vi "Tip Shaper_plus_plus.vi"() -> ()   [LabVIEW 2014]
doc: "Performs a configurable bias/Z sequence that can help to shape a STM tip.\n\n- Nanonis Programming Interface -"
uses:
  <userlib>/Nanonis Prog Interface V5/Nanonis Prog Interface.lvlib
panel:
  in  "Clear Markers":bool
  in  "Current Gain":u16(ring)=13 items=["HS 10^5", "HS 10^6", "HS 10^7", "HS 10^8", "HS 10^9", "HS 10^10", "HS 10^11", "LN 10^3", "LN 10^4", "LN 10^5", "LN 10^6", "LN 10^7", "LN 10^8", "LN 10^9"]
  in  "Bias value":dbl=0.02 format="%.3p"
  in  "Change Bias":bool=TRUE
  in  "Switch Gain":bool=TRUE
  in  "Draw":bool=TRUE
  in  "Lift Time 1":dbl=0.2 min=0.02 max=600.0 format="%.2p"
  out "Bias (V)":sgl=-2.0 format="%_5p"
  in  "Feedback":bool=TRUE
  out "oStartSequence":refnum<k4>
  in  "cleanTip":bool
  out "allQuit":bool=TRUE
  in  "quit":bool=TRUE
  out "oUpdateDisplay":refnum<k4>
  in  "End Wait Time":dbl=0.1 format="%.2p"
  in  "Lifting Bias":dbl=2.0 format="%.3p"
  in  "Lift Time 2":dbl=1.0 min=0.02 max=600.0 format="%.2p"
  in  "Lift Height":dbl=5e-09 format="%.2p"
  in  "Switch Off Delay":dbl=0.05 format="%.2p"
  in  "Bias Settling Time":dbl=0.09999999999999999 format="%.2p"
  in  "TipLift":dbl=-2e-10 format="%.2p"
  out "Z Graph":cluster{dbl[], dbl[]}[](graph)=[{[0.0, 0.10999999999999999, 0.10999999999999999, 0.20999999999999996, 0.41, 0.41, 0.51, 1.51, 1.51, 1.61], [0.0, 0.0, 0.0, 0.0, -2e-10, -2e-10, -2e-10, 5e-09, 5e-09, 5e-09]}, {[0.0, 0.10999999999999999, 0.10999999999999999, 0.20999999999999996, 0.41, 0.41, 0.51, 1.51, 1.51, 1.61], [-2.0, -2.0, 1.0, 1.0, 1.0, 2.0, 2.0, 2.0, -2.0, -2.0]}]
  # "Parameters"
  # "Internal Variables"
  # "s"
  # "V"
  # "m"
  # "s"
  # "V"
  # "s"
  # "m"
  # "s"
  # "s"
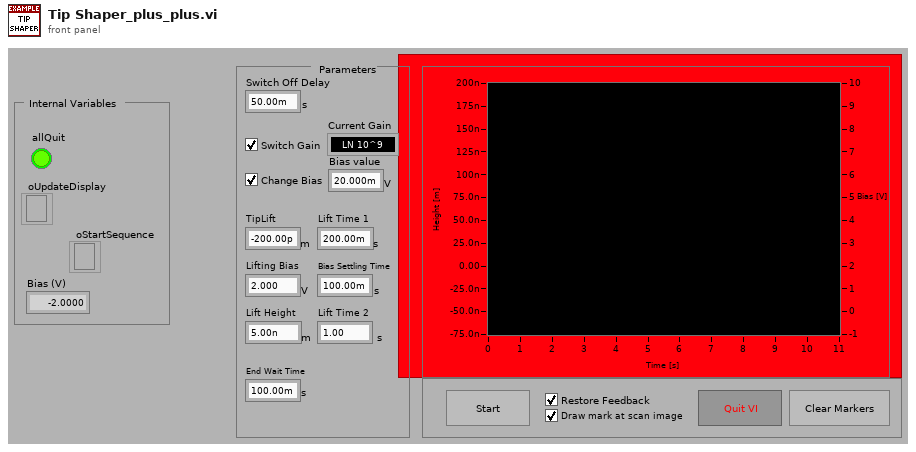
[diagram p1: front panel]
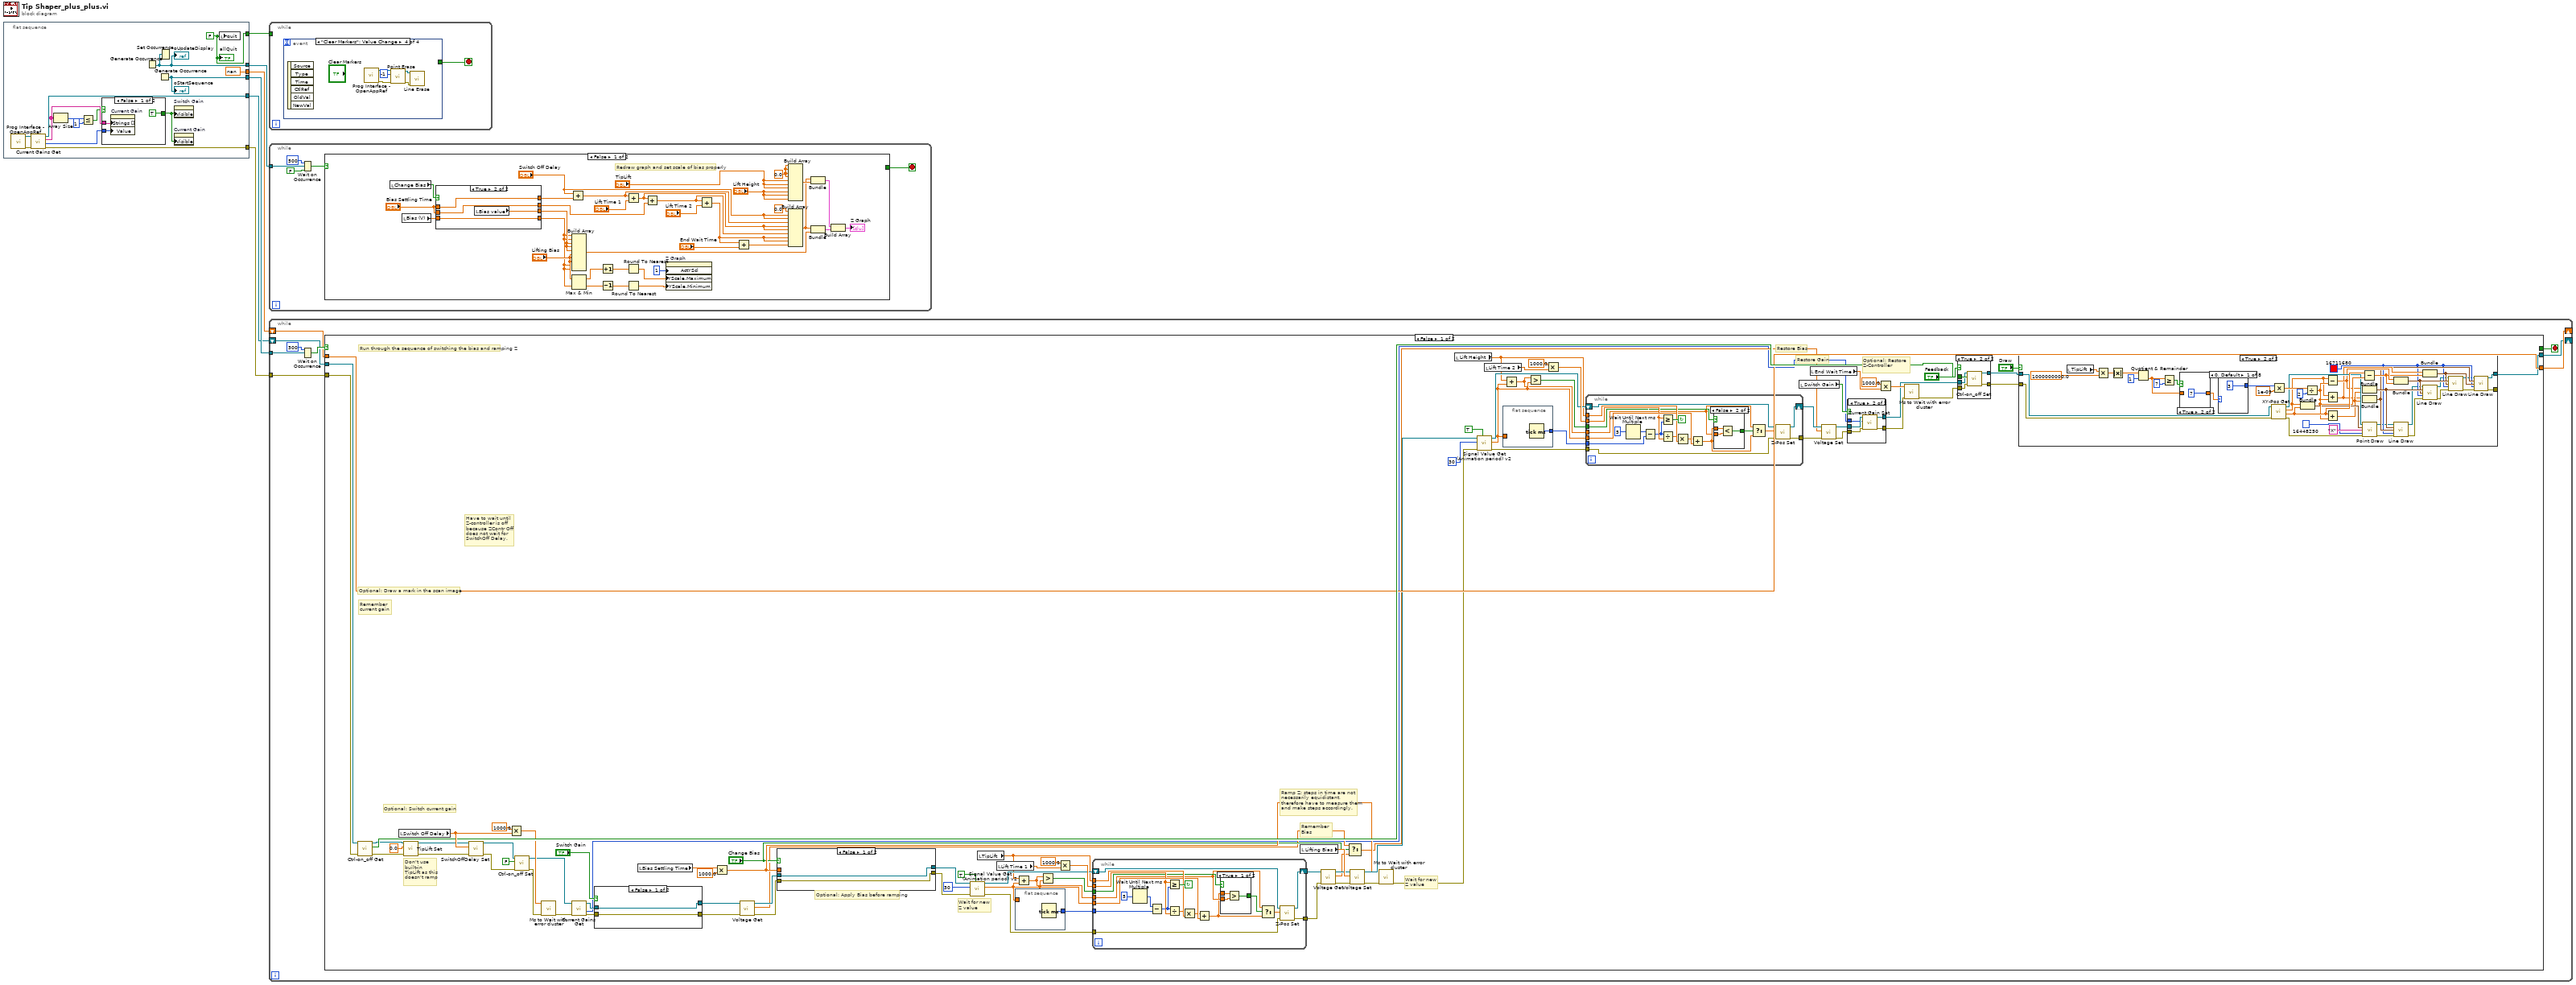
[diagram p0: block diagram]
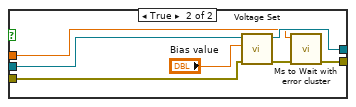
[diagram p3: hidden frame]
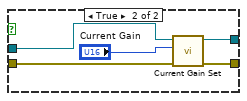
[diagram p4: hidden frame]
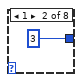
[diagram p6: hidden frame]
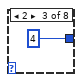
[diagram p7: hidden frame]
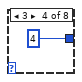
[diagram p8: hidden frame]
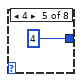
[diagram p9: hidden frame]
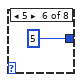
[diagram p10: hidden frame]
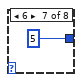
[diagram p11: hidden frame]
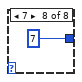
[diagram p12: hidden frame]
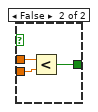
[diagram p14: hidden frame]
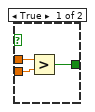
[diagram p16: hidden frame]
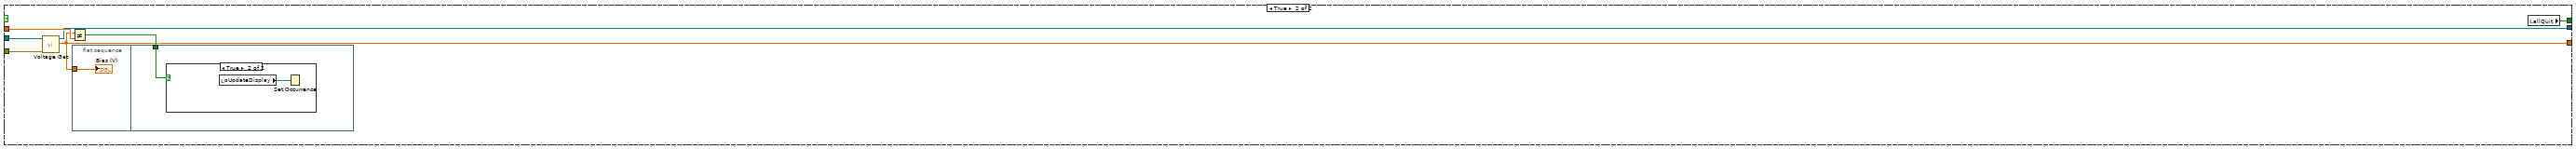
[diagram p17: hidden frame]
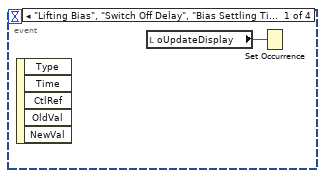
[diagram p19: hidden frame]
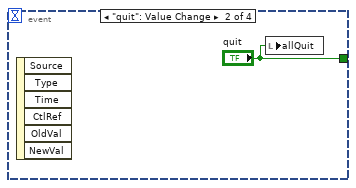
[diagram p20: hidden frame]
diagram:
  n1 = flat-sequence {
    tunnel: [w18] -> w6
    tunnel: [w20] -> w5
    tunnel: [w19] -> w4
    tunnel: [w12] -> w3
    tunnel: [sgl nan ("Bias (V)")] -> w2
    tunnel: [w13] -> w1
    frame #0 {
      w18 = FALSE ("allQuit")
      n2 = call <userlib>:"Prog Interface - OpenAppRef.vi"() -> ("Error out"=w14:errorcluster, "Application reference"=w15:refnum<vi>)  [unwired: 6 in]
      n3 = call <userlib>:"Current Gains Get.vi"("Error in (no error)"=w14, "Application ref in"=w15) -> ("Error out"=w12:errorcluster, "Selected Gain"=w16:u16, "Gains"=w11:string[], "Application ref out"=w13:refnum<vi>)  [unwired: 6 in]
      n4 = Array Size(array=w11) -> (size(s)=w10:i32)
      n5 = Less Or Equal?(x=w10, y=1) -> (x <= y?=w8:bool)
      n6 = case shown="False" w8 {
        tunnel: w16 -> [w23 _]
        tunnel: w11 -> [w22 _]
        tunnel: [TRUE FALSE] -> w7
        frame False {
          n7 = property on="Current Gain" class="Ring (strict)"("Strings []"=w22, "Value"=w23) -> ()  [unwired: 2 in, 2 out]
        }
        frame True {
        }
      }
      n8 = Generate Occurrence() -> (w20:refnum<k4>)
      "oUpdateDisplay" <- w20
      n9 = Generate Occurrence() -> (w19:refnum<k4>)
      "oStartSequence" <- w19
      n10 = Set Occurrence(w20) -> ()
      n11 = property on="Switch Gain" class="Bool (strict)"("Visible"=w7) -> ()  [unwired: 2 in, 2 out]
      n12 = property on="Current Gain" class="Ring (strict)"("Visible"=w7) -> ()  [unwired: 2 in, 2 out]
      n13 = local write "quit"(w18) -> ()
      "allQuit" <- w18
    }
  }
  n14 = while {
    tunnel: w6 -> [_]
    stop <- w25 stop-if-true
    n15 = event shown="[3] \"Clear Markers\": Value Change" {
      selector: _ -> [_ _ _ _]
      dyn-events: _ -> [_ _ _ _]
      timeout: _ -> [_ _ _ _]
      tunnel: [_ "quit" _ _] -> w25
      event "Lifting Bias", "Switch Off Delay", "Bias Settling Time", "Lift Time 2", "Lift Height", "End Wait Time", "TipLift", "Lift Time 1", "Change Bias", "Bias value": Value Change {
        n16 = event-data() -> ()  [unwired: 1 in, 5 out]
        n17 = local read "oUpdateDisplay"() -> (w26:refnum<k4>)
        n18 = Set Occurrence(w26) -> ()
      }
      event "quit": Value Change {
        n19 = event-data() -> ()  [unwired: 1 in, 6 out]
        n20 = local write "allQuit"("quit") -> ()
      }
      event "cleanTip": Value Change {
        n21 = event-data() -> ()  [unwired: 1 in, 6 out]
        n22 = local read "oStartSequence"() -> (w28:refnum<k4>)
        n23 = Set Occurrence(w28) -> ()
      }
      event "Clear Markers": Value Change {
        n24 = event-data() -> ()  [unwired: 1 in, 6 out]
        n25 = call <userlib>:"Prog Interface - OpenAppRef.vi"() -> ("Error out"=w33:errorcluster, "Application reference"=w32:refnum<vi>)  [unwired: 6 in]
        n26 = call <userlib>:"Point Erase.vi"("Application ref in"=w32, "Point index (-1=All points)"=-1, "error in (no error)"=w33) -> ("Application ref out"=w30:refnum<vi>, "error out"=w29:errorcluster)  [unwired: 11 in]
        n27 = call <userlib>:"Line Erase.vi"("Application ref in"=w30, "error in (no error)"=w29) -> ()  [unwired: 12 in, 2 out]
      }
    }
  }
  n28 = while {
    tunnel: w5 -> [w34]
    stop <- w37 stop-if-true
    n29 = Wait on Occurrence(1:FALSE ("ignore previous (T)"), 2:w34, 3:500 ("ms timeout (-1)")) -> (0:w38:bool)
    n30 = case shown="False" w38 {
      tunnel: [_ w80] -> w37
      frame False {
        w48 = 0.0 ("new element/subarray")
        # "Redraw graph and set scale of bias properly"
        n31 = local read "Change Bias"() -> (w41:bool)
        n32 = local read "Bias (V)"() -> (w42:sgl)
        n33 = case shown="True" w41 {
          tunnel: [0.0 ("Bias Settling Time (s)") w79] -> w45
          tunnel: "Bias Settling Time" -> [_ w79]
          tunnel: [w73 w76] -> w40
          tunnel: [w75 w78] -> w44
          tunnel: "Bias Settling Time" -> [w75 w78]
          tunnel: [w73 w77] -> w39
          tunnel: w42 -> [w73 w77]
          frame False {
          }
          frame True {
            n34 = local read "Bias value"() -> (w76:dbl)
          }
        }
        n35 = Add(x="Switch Off Delay", y=w45) -> (x+y=w46:dbl)
        n36 = Build Array(w39, w39, w40, w40, w40, "Lifting Bias", "Lifting Bias", "Lifting Bias", w39, w39) -> (w61:dbl[])
        n37 = Max & Min(x="Lifting Bias", y=w39) -> (max(x,y)=w57:dbl, min(x,y)=w56:dbl)
        n38 = Increment(x=w57) -> (x+1=w58:dbl)
        n39 = Decrement(x=w56) -> (x-1=w55:dbl)
        n40 = Add(x=w46, y="Lift Time 1") -> (x+y=w50:dbl)
        n41 = Round To Nearest(number=w58) -> (nearest integer value=w59:dbl)
        n42 = Round To Nearest(number=w55) -> (nearest integer value=w60:dbl)
        n43 = Add(x=w50, y=w44) -> (x+y=w51:dbl)
        n44 = property on="Z Graph" class="XYGraph (strict)"("ActYScl"=1 ("Active Y Scale"), "YScale.Maximum"=w59, "YScale.Minimum"=w60) -> ()  [unwired: 2 in, 2 out]
        n45 = Add(x=w51, y="Lift Time 2") -> (x+y=w69:dbl)
        n46 = Add(x=w69, y="End Wait Time") -> (x+y=w68:dbl)
        n47 = Build Array(w48, w48, w48, w48, "TipLift", "TipLift", "TipLift", "Lift Height", "Lift Height", "Lift Height") -> (w66:dbl[])
        n48 = Build Array(0.0 ("new element/subarray"), "Switch Off Delay", "Switch Off Delay", w46, w50, w50, w51, w69, w69, w68) -> (w62:dbl[])
        n49 = Bundle(w62, w66) -> (w65:cluster{dbl[], dbl[]})  [unwired: 1 in]
        n50 = Bundle(w62, w61) -> (w64:cluster{dbl[], dbl[]})  [unwired: 1 in]
        n51 = Build Array(w65, w64) -> (→"Z Graph":cluster{dbl[], dbl[]}[])
      }
      frame True {
        n52 = local read "allQuit"() -> (w80:bool)
      }
    }
  }
  n53 = while {
    tunnel: w4 -> [w87]
    tunnel: w3 -> [w85]
    shift-right: [w83] -> _
    shift-left: w2 -> [w84]
    shift-right: [w81] -> _
    shift-left: w1 -> [w82]
    stop <- w86 stop-if-true
    n54 = Wait on Occurrence(2:w87, 3:300 ("ms timeout (-1)")) -> (0:w88:bool)  [unwired: 1 in]
    n55 = case shown="False" w88 {
      tunnel: [_ w315] -> w86
      tunnel: w85 -> [w153 w311]
      tunnel: w84 -> [w150 w313]
      tunnel: [w150 w312] -> w83
      tunnel: w82 -> [w135 w310]
      tunnel: [w120 w309] -> w81
      frame False {
        # "Ramp Z: steps in time are not necessarily equidistant, therefore have to measure them and make steps accordingly."
        # "Optional: Draw a mark in the scan image"
        # "Optional: Apply Bias before ramping"
        # "Remember Bias"
        # "Optional: Switch current gain"
        # "Remember current gain"
        # "Restore Bias"
        # "Optional: Restore Z-Controller"
        # "Restore Gain"
        # "Don't use built-in TipLift as this doesn't ramp"
        # "Wait for new Z value"
        # "Have to wait until Z-controller is off because ZContr Off does not wait for SwitchOff Delay."
        # "Wait for new Z value"
        # "Run through the sequence of switching the bias and ramping Z"
        n56 = call <userlib>:"Ctrl-on_off Get.vi"("error in (no error)"=w153, "Application ref in"=w135) -> ("error out"=w152:errorcluster, "Z-Controller on/off status"=w151:bool, "Application ref out"=w134:refnum<vi>)  [unwired: 7 in]
        n57 = local read "Switch Off Delay"() -> (w161:dbl)
        n58 = call <userlib>:"TipLift Set.vi"("error in (no error)"=w152, "TipLift (m)"=sgl 0.0, "Application ref in"=w134) -> ("error out"=w172:errorcluster, "Application ref out"=w133:refnum<vi>)  [unwired: 7 in]
        n59 = call <userlib>:"SwitchOffDelay Set.vi"("error in (no error)"=w172, "Switch off Delay (s)"=w161, "Application ref in"=w133) -> ("error out"=w141:errorcluster, "Application ref out"=w132:refnum<vi>)  [unwired: 7 in]
        n60 = Multiply(x=1000.0, y=w161) -> (x*y=w149:dbl)
        n61 = call <userlib>:"Ctrl-on_off Set.vi"("error in (no error)"=w141, "Z Controller ON/OFF"=FALSE, "Application ref in"=w132) -> ("error out"=w157:errorcluster, "Application ref out"=w107:refnum<vi>)  [unwired: 7 in]
        n62 = call <userlib>:"Ms to Wait with error cluster.vi"("error in (no error)"=w157, "milliseconds to wait"=w149) -> ("error out"=w105:errorcluster)  [unwired: 4 in, 1 out]
        n63 = call <userlib>:"Current Gains Get.vi"("Error in (no error)"=w105, "Application ref in"=w107) -> ("Error out"=w104:errorcluster, "Selected Gain"=w98:u16, "Application ref out"=w106:refnum<vi>)  [unwired: 6 in, 1 out]
        n64 = case shown="False" "Switch Gain" {
          tunnel: w106 -> [w190 w195]
          tunnel: w104 -> [w189 w194]
          tunnel: [w190 w192] -> w112
          tunnel: [w189 w193] -> w110
          frame False {
          }
          frame True {
            n65 = call <userlib>:"Current Gain Set.vi"("Error in (no error)"=w194, "Gain index"="Current Gain", "Application ref in"=w195) -> ("Error out"=w193:errorcluster, "Application ref out"=w192:refnum<vi>)  [unwired: 7 in]
          }
        }
        n66 = local read "Bias Settling Time"() -> (w159:dbl)
        n67 = Multiply(x=w159, y=1000.0) -> (x*y=w116:dbl)
        n68 = call <userlib>:"Voltage Get.vi"("error in (no error)"=w110, "Application ref in"=w112) -> ("error out"=w109:errorcluster, "Bias (V)"=w108:sgl, "Application ref out"=w111:refnum<vi>)  [unwired: 7 in]
        n69 = case shown="False" "Change Bias" {
          tunnel: w111 -> [w181 w183]
          tunnel: [w181 w187] -> w118
          tunnel: w109 -> [w180 w182]
          tunnel: [w180 w186] -> w117
          tunnel: w116 -> [_ w185]
          frame False {
          }
          frame True {
            n70 = call <userlib>:"Voltage Set.vi"("Error in (no error)"=w182, "Bias (V)"="Bias value", "Application ref in"=w183) -> ("Error out"=w188:errorcluster, "Application ref out"=w187:refnum<vi>)  [unwired: 7 in]
            n71 = call <userlib>:"Ms to Wait with error cluster.vi"("error in (no error)"=w188, "milliseconds to wait"=w185) -> ("error out"=w186:errorcluster)  [unwired: 4 in, 1 out]
          }
        }
        n72 = call <userlib>:"Signal Value Get (Animation period) v2.vi"("Wait for newest data (F=False)"=TRUE ("Wait for newest data (F)"), "error in (no error)"=w117, "Signal index (0-79)"=i8 30 ("Signal index (0-23)"), "Application ref in"=w118) -> ("error out"=w144:errorcluster, "Signal value"=w95:sgl, "Application ref out"=w130:refnum<vi>)  [unwired: 4 in]
        n73 = local read "TipLift"() -> (w97:dbl)
        n74 = local read "Lift Time 1"() -> (w139:dbl)
        n75 = flat-sequence {
          tunnel: [w250] -> w143
          tunnel: w95 -> [_]
          frame #0 {
            n76 = Tick Count (ms)() -> (millisecond timer value=w250:u32)
          }
        }
        n77 = Add(x=w97, y=w95) -> (x+y=w96:dbl)
        n78 = Greater?(x=w96, y=w95) -> (0:w94:bool)
        n79 = Multiply(x=1000.0, y=w139) -> (x*y=w138:dbl)
        n80 = while {
          tunnel: w143 -> [w269]
          tunnel: w97 -> [w267]
          tunnel: [w266] -> w137
          tunnel: w95 -> [w262]
          tunnel: w144 -> [w263]
          tunnel: w138 -> [w260]
          shift-right: [w256] -> w129
          shift-left: w130 -> [w257]
          tunnel: w96 -> [w253]
          tunnel: w94 -> [w255]
          stop <- w268 continue-if-true
          n81 = Wait Until Next ms Multiple(millisecond multiple=u32 5) -> (millisecond timer value=w259:u32)
          n82 = Subtract(x=w259, y=w269) -> (x-y=w258:u32)
          n83 = Greater Or Equal?(x=w260, y=w258) -> (x >= y?=w268:bool)
          n84 = Divide(x=w258, y=w260) -> (x/y=w264:dbl)
          n85 = Multiply(x=w264, y=w267) -> (x*y=w261:dbl)
          n86 = Add(x=w261, y=w262) -> (x+y=w252:dbl)
          n87 = case shown="True" w255 {
            tunnel: w252 -> [w272 w275]
            tunnel: w253 -> [w271 w274]
            tunnel: [w270 w273] -> w254
            frame True {
              n88 = Greater?(x=w272, y=w271) -> (0:w270:bool)
            }
            frame False {
              n89 = Less?(x=w275, y=w274) -> (x < y?=w273:bool)
            }
          }
          n90 = Select(t=w253, s=w254, f=w252) -> (s? t:f=w251:dbl)
          n91 = call <userlib>:"Z-Pos Set.vi"("error in (no error)"=w263, "Z position (m)"=w251, "Application ref in"=w257) -> ("error out"=w266:errorcluster, "Application ref out"=w256:refnum<vi>)  [unwired: 7 in]
        }
        n92 = local read "Lifting Bias"() -> (w171:dbl)
        n93 = call <userlib>:"Voltage Get.vi"("error in (no error)"=w137, "Application ref in"=w129) -> ("error out"=w136:errorcluster, "Bias (V)"=w114:sgl, "Application ref out"=w128:refnum<vi>)  [unwired: 7 in]
        n94 = Select(t=w108, s="Change Bias", f=w114) -> (s? t:f=w113:sgl)
        n95 = call <userlib>:"Voltage Set.vi"("Error in (no error)"=w136, "Bias (V)"=w171, "Application ref in"=w128) -> ("Error out"=w156:errorcluster, "Application ref out"=w124:refnum<vi>)  [unwired: 7 in]
        n96 = call <userlib>:"Ms to Wait with error cluster.vi"("error in (no error)"=w156, "milliseconds to wait"=w116) -> ("error out"=w148:errorcluster)  [unwired: 4 in, 1 out]
        n97 = local read "Lift Height"() -> (w93:dbl)
        n98 = call <userlib>:"Signal Value Get (Animation period) v2.vi"("Wait for newest data (F=False)"=TRUE ("Wait for newest data (F)"), "error in (no error)"=w148, "Signal index (0-79)"=i8 30 ("Signal index (0-23)"), "Application ref in"=w124) -> ("error out"=w147:errorcluster, "Signal value"=w92:sgl, "Application ref out"=w126:refnum<vi>)  [unwired: 4 in]
        n99 = local read "Lift Time 2"() -> (w169:dbl)
        n100 = flat-sequence {
          tunnel: [w276] -> w165
          tunnel: w92 -> [_]
          frame #0 {
            n101 = Tick Count (ms)() -> (millisecond timer value=w276:u32)
          }
        }
        n102 = Add(x=w93, y=w92) -> (x+y=w90:dbl)
        n103 = Greater?(x=w90, y=w92) -> (0:w91:bool)
        n104 = Multiply(x=1000.0, y=w169) -> (x*y=w158:dbl)
        n105 = while {
          tunnel: w165 -> [w302]
          tunnel: w93 -> [w300]
          tunnel: [w299] -> w167
          tunnel: w92 -> [w295]
          tunnel: w147 -> [w296]
          tunnel: w158 -> [w293]
          shift-right: [w289] -> w125
          shift-left: w126 -> [w290]
          tunnel: w91 -> [w288]
          tunnel: w90 -> [w285]
          stop <- w301 continue-if-true
          n106 = Wait Until Next ms Multiple(millisecond multiple=u32 5) -> (millisecond timer value=w292:u32)
          n107 = Subtract(x=w292, y=w302) -> (x-y=w291:u32)
          n108 = Greater Or Equal?(x=w293, y=w291) -> (x >= y?=w301:bool)
          n109 = Divide(x=w291, y=w293) -> (x/y=w297:dbl)
          n110 = Multiply(x=w297, y=w300) -> (x*y=w294:dbl)
          n111 = Add(x=w294, y=w295) -> (x+y=w286:dbl)
          n112 = case shown="False" w288 {
            tunnel: w286 -> [w305 w308]
            tunnel: w285 -> [w304 w307]
            tunnel: [w303 w306] -> w287
            frame True {
              n113 = Greater?(x=w305, y=w304) -> (0:w303:bool)
            }
            frame False {
              n114 = Less?(x=w308, y=w307) -> (x < y?=w306:bool)
            }
          }
          n115 = Select(t=w285, s=w287, f=w286) -> (s? t:f=w284:dbl)
          n116 = call <userlib>:"Z-Pos Set.vi"("error in (no error)"=w296, "Z position (m)"=w284, "Application ref in"=w290) -> ("error out"=w299:errorcluster, "Application ref out"=w289:refnum<vi>)  [unwired: 7 in]
        }
        n117 = local read "Switch Gain"() -> (w103:bool)
        n118 = local read "End Wait Time"() -> (w163:dbl)
        n119 = call <userlib>:"Voltage Set.vi"("Error in (no error)"=w167, "Bias (V)"=w113, "Application ref in"=w125) -> ("Error out"=w100:errorcluster, "Application ref out"=w102:refnum<vi>)  [unwired: 7 in]
        n120 = case shown="True" w103 {
          tunnel: w102 -> [w174 w179]
          tunnel: [w174 w178] -> w101
          tunnel: w100 -> [w173 w177]
          tunnel: [w173 w176] -> w99
          tunnel: w98 -> [_ w175]
          frame False {
          }
          frame True {
            n121 = call <userlib>:"Current Gain Set.vi"("Error in (no error)"=w177, "Gain index"=w175, "Application ref in"=w179) -> ("Error out"=w176:errorcluster, "Application ref out"=w178:refnum<vi>)  [unwired: 7 in]
          }
        }
        n122 = Multiply(x=1000.0, y=w163) -> (x*y=w154:dbl)
        n123 = call <userlib>:"Ms to Wait with error cluster.vi"("error in (no error)"=w99, "milliseconds to wait"=w154) -> ("error out"=w155:errorcluster)  [unwired: 4 in, 1 out]
        n124 = case shown="True" "Feedback" {
          tunnel: w155 -> [w277 w283]
          tunnel: w151 -> [_ w282]
          tunnel: w101 -> [w278 w281]
          tunnel: [w278 w280] -> w122
          tunnel: [w277 w279] -> w121
          frame False {
          }
          frame True {
            n125 = call <userlib>:"Ctrl-on_off Set.vi"("error in (no error)"=w283, "Z Controller ON/OFF"=w282, "Application ref in"=w281) -> ("error out"=w279:errorcluster, "Application ref out"=w280:refnum<vi>)  [unwired: 7 in]
          }
        }
        n126 = case shown="True" "Draw" {
          tunnel: w122 -> [w197 w239]
          tunnel: w121 -> [w196 w238]
          tunnel: [w197 w200] -> w120
          tunnel: [w196 w201] -> _
          frame False {
          }
          frame True {
            w210 = u32 16711680
            n127 = local read "TipLift"() -> (w227:dbl)
            n128 = Multiply(x=w227, y=1000000000.0) -> (x*y=w228:dbl)
            n129 = Absolute Value(x=w228) -> (abs(x)=w231:dbl)
            n130 = Quotient & Remainder(x=w231, y=1) -> (floor(x/y)=w233:dbl)  [unwired: 1 out]
            n131 = Greater Or Equal?(x=w233, y=7) -> (x >= y?=w232:bool)
            n132 = case shown="True" w232 {
              tunnel: [w248 7] -> w199
              tunnel: w233 -> [w248 _]
              frame False {
              }
              frame True {
              }
            }
            n133 = case shown="0, Default" w199 {
              tunnel: [3 3 4 4 4 5 5 7] -> w235
              frame 0, Default {
              }
              frame 1 {
              }
              frame 2 {
              }
              frame 3 {
              }
              frame 4 {
              }
              frame 5 {
              }
              frame 6 {
              }
              frame 7 {
              }
            }
            n134 = call <userlib>:"XY-Pos Get.vi"("error in (no error)"=w238, "Application ref in"=w239) -> ("error out"=w219:errorcluster, "Y (m)"=w225:sgl, "X (m)"=w223:sgl, "Application ref out"=w220:refnum<vi>)  [unwired: 5 in]
            n135 = Multiply(x=w235, y=1e-09) -> (x*y=w236:dbl)
            n136 = Bundle("X (m)"=w223, "Y (m)"=w225) -> (w222:cluster{"X (m)":sgl, "Y (m)":sgl})  [unwired: 1 in]
            n137 = Divide(x=w236, y=2) -> (x/y=w224:dbl)
            n138 = Subtract(x=w223, y=w224) -> (x-y=w216:dbl)
            n139 = Add(x=w223, y=w224) -> (x+y=w214:dbl)
            n140 = Add(x=w225, y=w224) -> (x+y=w218:dbl)
            n141 = Subtract(x=w225, y=w224) -> (x-y=w213:dbl)
            n142 = Bundle(w216, w218) -> (w217:cluster{dbl, dbl})  [unwired: 1 in]
            n143 = Bundle(w214, w218) -> (w212:cluster{dbl, dbl})  [unwired: 1 in]
            n144 = call <userlib>:"Point Draw.vi"("Application ref in"=w220, "Point Coordinates"=w222, "Text"="X", "Color"=u32 16448250, "error in (no error)"=w219) -> ("Application ref out"=w209:refnum<vi>, "error out"=w205:errorcluster)  [unwired: 9 in]
            n145 = Bundle(w216, w213) -> (w215:cluster{dbl, dbl})  [unwired: 1 in]
            n146 = call <userlib>:"Line Draw.vi"("Application ref in"=w209, "Start Point Coordinates"=w217, "End Point Coordinates"=w212, "Color"=w210, "error in (no error)"=w205) -> ("Application ref out"=w208:refnum<vi>, "error out"=w204:errorcluster)  [unwired: 9 in]
            n147 = Bundle(w214, w213) -> (w211:cluster{dbl, dbl})  [unwired: 1 in]
            n148 = call <userlib>:"Line Draw.vi"("Application ref in"=w208, "Start Point Coordinates"=w217, "End Point Coordinates"=w215, "Color"=w210, "error in (no error)"=w204) -> ("Application ref out"=w207:refnum<vi>, "error out"=w203:errorcluster)  [unwired: 9 in]
            n149 = call <userlib>:"Line Draw.vi"("Application ref in"=w207, "Start Point Coordinates"=w215, "End Point Coordinates"=w211, "Color"=w210, "error in (no error)"=w203) -> ("Application ref out"=w206:refnum<vi>, "error out"=w202:errorcluster)  [unwired: 9 in]
            n150 = call <userlib>:"Line Draw.vi"("Application ref in"=w206, "Start Point Coordinates"=w212, "End Point Coordinates"=w211, "Color"=w210, "error in (no error)"=w202) -> ("Application ref out"=w200:refnum<vi>, "error out"=w201:errorcluster)  [unwired: 9 in]
          }
        }
      }
      frame True {
        n151 = call <userlib>:"Voltage Get.vi"("error in (no error)"=w311, "Application ref in"=w310) -> ("Bias (V)"=w312:sgl, "Application ref out"=w309:refnum<vi>)  [unwired: 7 in, 1 out]
        n152 = Not Equal?(x=w312, y=w313) -> (x != y?=w314:bool)
        n153 = flat-sequence {
          tunnel: w312 -> [w316]
          tunnel: w314 -> [w317]
          frame #0 {
            "Bias (V)" <- w316
          }
          frame #1 {
            n154 = case shown="True" w317 {
              frame False {
              }
              frame True {
                n155 = local read "oUpdateDisplay"() -> (w318:refnum<k4>)
                n156 = Set Occurrence(w318) -> ()
              }
            }
          }
        }
        n157 = local read "allQuit"() -> (w315:bool)
      }
    }
  }
